vi "Chirp Pattern (CDB).vi"(8 "f2":dbl=0.05, 9 "f1":dbl=-0.05, 10 "amplitude":dbl=1.0, 11 "samples":i32=1024) -> (3 "complex chirp":cdb[](array[numeric]))   [LabVIEW 2013, in "rf-utils.lvlib"]
uses:
  rf-utils.lvlib
  <vilib>/Analysis/1siggen.llb/Ramp Pattern by Samples.vi
  <vilib>/Analysis/NI_AALBase.lvlib
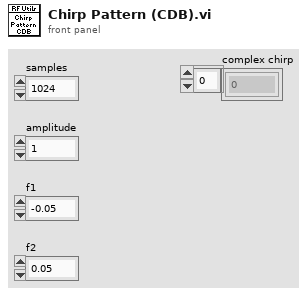
[diagram p1: front panel]
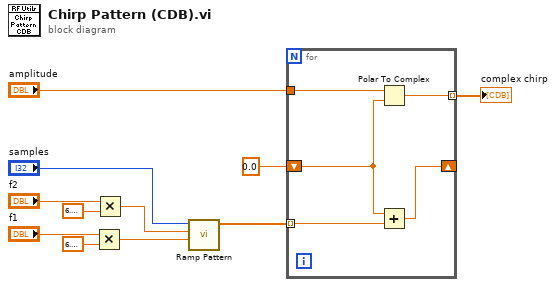
[diagram p0: block diagram]
diagram:
  n1 = Multiply(x="f1", y=6.283185307179586) -> (x*y=w3:dbl)
  n2 = Multiply(x="f2", y=6.283185307179586) -> (x*y=w4:dbl)
  n3 = call-poly <vilib>:"Ramp Pattern.vi"("start"=w3, "end"=w4, "samples"="samples") -> ("Ramp Pattern"=w2:dbl[])  [unwired: 7 in, 1 out]
  n4 = for {
    tunnel: "amplitude" -> [w16]
    tunnel: [w15] -> w5 mode=indexing
    shift-right: [w14] -> _
    shift-left: 0.0 -> [w13]
    tunnel: w2 -> [w12] mode=indexing
    n5 = Polar To Complex(1:w13, 2:w16) -> (0:w15:cdb)
    n6 = Add(x=w13, y=w12) -> (x+y=w14:dbl)
  }
  "complex chirp" <- w5
